vi "Send Configure Channel.vi"(2 "vertical range (10.0 V)":dbl[unit]=10.0 format="%.3f", 4 "vertical coupling (DC)":i32(ring)=1 items=["AC", "DC", "GND"], 5 "vertical offset (0.0 V)":dbl[unit] format="%.3f", 6 "probe attenuation (1:1.0)":dbl=1.0 format="%.3f", 7 "Message Priority (Normal)":T1=enum."Normal", 8 "error in (no error)":errorcluster, 9 "channel name (\"CHANNEL1\")":string="CHANNEL1", 10 "channel enabled (True)":bool=TRUE, 11 "Message Enqueuer":refnum<class "Message Enqueuer.lvclass">) -> (0 "error out":errorcluster, 3 "Message Enqueuer out":refnum<class "Message Enqueuer.lvclass">)   [LabVIEW 2016, in "CS++Scope.lvlib" / "Configure Channel Msg.lvclass"]
doc: "Sends the <B>CS++Scope.lvlib:Configure Channel Msg.lvclass</B> message.\n\n<B>CS++Scope.lvlib:CS++Scope.lvclass:Configure Channel.vi</B> Description:\n\nThis VI configures the most commonly configured properties of the oscilloscope channel sub-system. These properties are the range, offset, coupling, probe attenuation, and whether the channel is enabled."
uses:
  Configure Channel Msg.lvclass
  <vilib>/ActorFramework/Message Enqueuer/Message Enqueuer.lvclass
  <vilib>/ActorFramework/Message Enqueuer/Message Priority.ctl
  C:/Program Files (x86)/National Instruments/LabVIEW 2016/vi.lib/ActorFramework/Message/Message.lvclass
  Configure Channel Msg.lvclass/Configure Channel Msg.ctl
  <vilib>/ActorFramework/Message Enqueuer/Message Enqueuer.lvclass/Message Enqueuer.ctl
  <vilib>/ActorFramework/Message Priority Queue/Priority Enqueue.vi
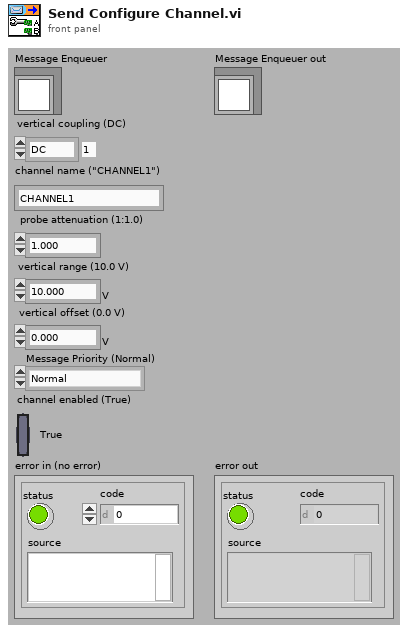
[diagram p1: front panel]
types:
  T1 = typedef "Actor Framework.lvlib/Message Enqueuer.lvclass/Message Priority.ctl" = enum16{"Low", "Normal", "High"}
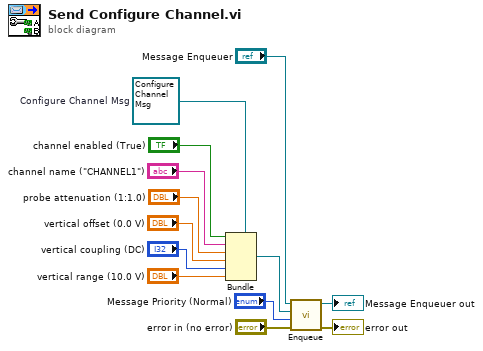
[diagram p0: block diagram]
diagram:
  w7 = refnum<class "Configure Channel Msg.lvclass"> refnum  # Configure Channel Msg
  n1 = Bundle(cluster=w7, "channel enabled (True)", "channel name (\"CHANNEL1\")", "probe attenuation (1:1.0)", "vertical offset (0.0 V)", "vertical coupling (DC)", "vertical range (10.0 V)") -> (w10:refnum<class "Configure Channel Msg.lvclass">)
  n2 = call <vilib>:"Enqueue.vi"("error in (no error)"="error in (no error)", "Message Priority (Normal)"="Message Priority (Normal)", "Message"=w10, "Message Enqueuer in"="Message Enqueuer") -> ("error out"=→"error out":errorcluster, "Message Enqueuer out"=→"Message Enqueuer out":refnum<class "Message Enqueuer.lvclass">)  [unwired: 6 in]
